vi "lockin - Set all f same.vi"(8 "error in (no error)":errorcluster, 11 "LockinDAQ":refnum<class "LockinDAQ.lvclass">) -> (0 "error out":errorcluster, 3 "LockinDAQ out":refnum<class "LockinDAQ.lvclass">)   [LabVIEW 2016, in "LockinDAQ.lvclass"]
uses:
  LockinDAQ.lvclass
  LockinDAQ.lvclass/LockinDAQ.ctl
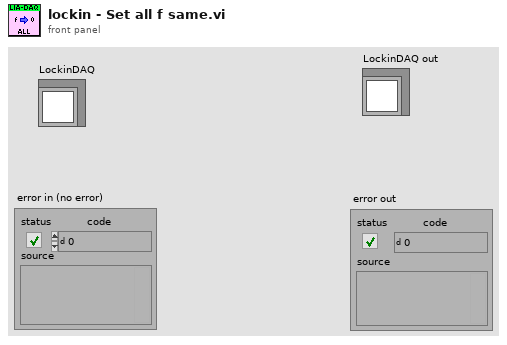
[diagram p1: front panel]
types:
  T1 = typedef "LockinDAQ.lvclass/AO-cluster.ctl" = cluster{"Ch":i32[], "Amp (V)":dbl[], "DC (V)":dbl[], "f (Hz)":dbl[], "Phase (°)":dbl[], "Function":T2[], "Sweep?":bool[]}
  T2 = typedef "LockinDAQ.lvclass/Function-enum.ctl" = enum16{"Sine", "Triangle", "Square", "Sawtooth"}
  T3 = typedef "LockinDAQ.lvclass/REF-cluster.ctl" = cluster{"Ch":i32[], " f (Hz)":dbl[], "Phase (°)":dbl[], "TC (s)":dbl[], "order":i32[]}
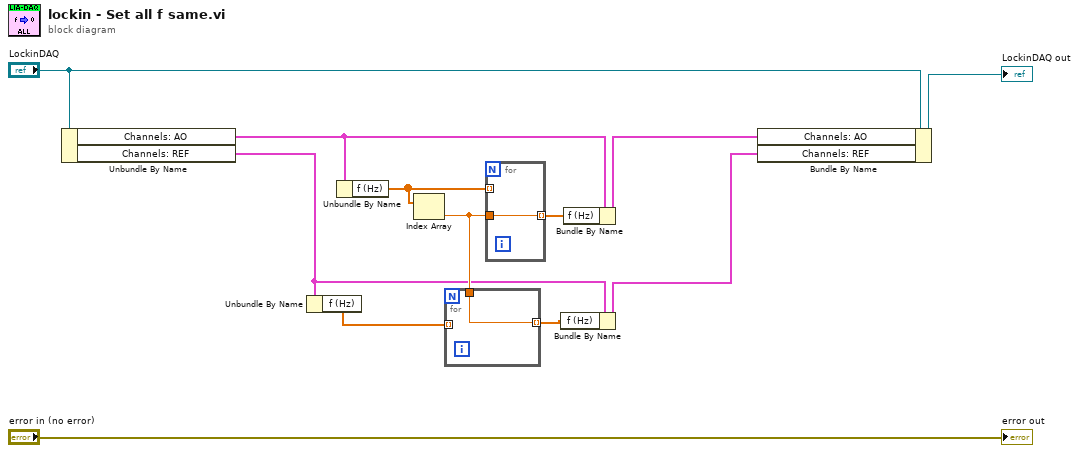
[diagram p0: block diagram]
diagram:
  n1 = Unbundle By Name("LockinDAQ") -> ("Channels: AO"=w2:T1, "Channels: REF"=w1:T3)
  n2 = Unbundle By Name(w1) -> ("f (Hz)"=w9:dbl[])
  n3 = Unbundle By Name(w2) -> ("f (Hz)"=w5:dbl[])
  n4 = Index Array(array=w5) -> (element=w7:dbl)  [unwired: 1 in]
  n5 = for {
    tunnel: w9 -> [_] mode=indexing
    tunnel: [w13] -> w8 mode=indexing
    tunnel: w7 -> [w13]
  }
  n6 = for {
    tunnel: w7 -> [w14]
    tunnel: [w14] -> w6 mode=indexing
    tunnel: w5 -> [_] mode=indexing
  }
  n7 = Bundle By Name(cluster=w1, "f (Hz)"=w8) -> (w4:T3)
  n8 = Bundle By Name(cluster=w2, "f (Hz)"=w6) -> (w3:T1)
  n9 = Bundle By Name(cluster="LockinDAQ", "Channels: AO"=w3, "Channels: REF"=w4) -> (→"LockinDAQ out":refnum<class "LockinDAQ.lvclass">)
  "error out" <- "error in (no error)"
